vi "LCD Print.vi"(0 "Arduino Resource":T1, 5 "Data":string, 7 "Base (String)":T3(ring), 11 "error out":errorcluster) -> (4 "Arduino Resource":T1, 15 "error out":errorcluster)   [LabVIEW 2015, in "LabVIEW Interface for Arduino.lvlib"]
doc: "Prints data of the specified type to the LCD screen."
uses:
  <vilib>/LabVIEW Interface for Arduino/LabVIEW Interface for Arduino.lvlib
  <vilib>/LabVIEW Interface for Arduino/Type Defs/Arduino Resource.ctl
  <vilib>/LabVIEW Interface for Arduino/Type Defs/Board Type.ctl
  <vilib>/LabVIEW Interface for Arduino/Type Defs/Command.ctl
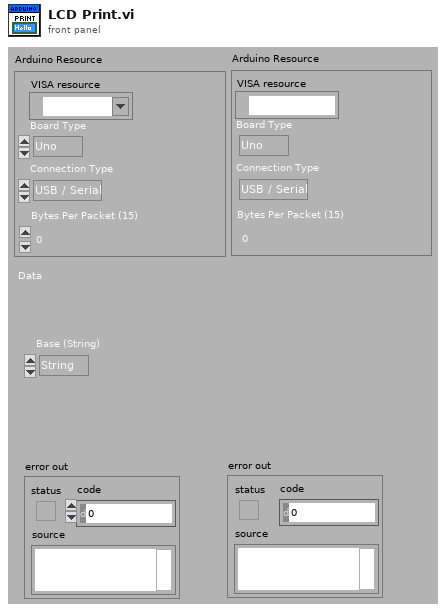
[diagram p1: front panel]
types:
  T1 = typedef "LabVIEW Interface for Arduino.lvlib/Arduino Resource.ctl" = cluster{"VISA resource":refnum<visa-resource-name>, "Board Type":T2, "Connection Type":enum8{"USB / Serial"}, "Bytes Per Packet (15)":u8}
  T2 = typedef "LabVIEW Interface for Arduino.lvlib/Board Type.ctl" = enum16{"Uno", "Dimuelanove w/Atmega 328", "Mega 2560"}
  T3 = enum8{"String", "Binary", "Decimal", "Octal", "Hexadecimal"}
  T4 = typedef "LabVIEW Interface for Arduino.lvlib/Command.ctl" = enum8{"setArduinoMode", "flushSerial", "setPinMode", "digitalWritePin", "digitalWritePort", "tone", "digitalReadPin", "digitalReadPort", "analogReadPin", "analogReadPort", "pwmWritePin", "pwmWritePort", "sevenSegment_Configure", "sevenSegment_Write", "I2C Init", "I2C Write", "I2C Read", "SPI Init", "SPI Set Bit Order", "SPI Set Clock Divider", "SPI Set Data Mode", "SPI Send / Receive", "SPI Close", "Servo Set Num Servos", "Servo Config Servo", "Servo Write Angle", "Servo Read Angle", "Servo Write Pulse Width", "Servo Read Pulse Width", "Servo Detach", "LCD Init", "LCD Set Size", "LCD Set Cursor Mode", "LCD Clear", "LCD Set Cursor Position", "LCD Print", "LCD Display Power", "LCD Scroll Display", "LCD Autoscroll", "LCD Print Direction", "LCD Create Custom Char", "LCD Print Custom Char", "contAcqOn", "contAcqOff", "getFirmwareVersion", "FiniteSampleStart"}
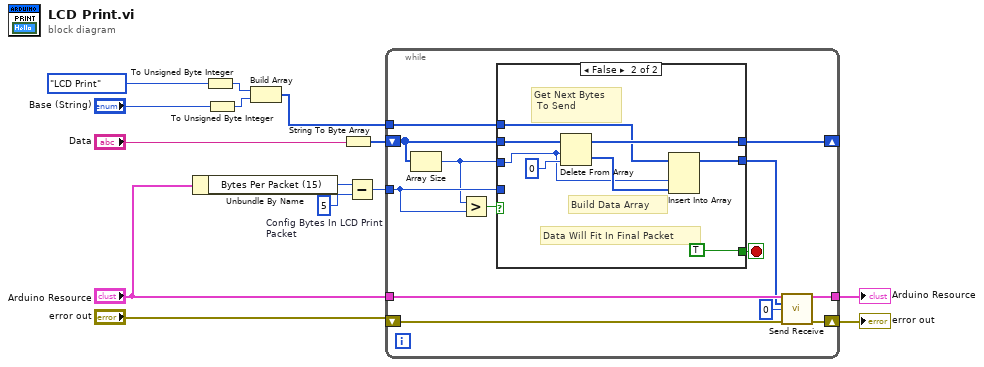
[diagram p0: block diagram]
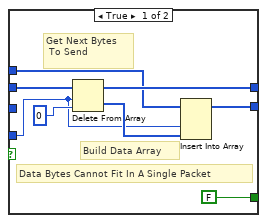
[diagram p2: hidden frame]
diagram:
  w6 = u8 5  # Config Bytes In LCD Print Packet
  n1 = Unbundle By Name("Arduino Resource") -> ("Bytes Per Packet (15)"=w2:u8)
  n2 = To Unsigned Byte Integer(number=Command."LCD Print" ("Command")) -> (unsigned 8bit integer=w10:u8)
  n3 = To Unsigned Byte Integer(number="Base (String)") -> (unsigned 8bit integer=w3:u8)
  n4 = Build Array(w10, w3) -> (w1:u8[])
  n5 = String To Byte Array(string="Data") -> (unsigned byte array=w5:u8[])
  n6 = Subtract(x=w2, y=w6) -> (x-y=w4:u8)
  n7 = while {
    tunnel: [w26] -> w13
    tunnel: "Arduino Resource" -> [w24]
    shift-right: [w27] -> w14
    shift-left: "error out" -> [w25]
    shift-right: [w22] -> _
    shift-left: w5 -> [w18]
    tunnel: w4 -> [w17]
    tunnel: w1 -> [w21]
    stop <- w15 stop-if-true
    n8 = Array Size(array=w18) -> (size(s)=w16:i32)
    n9 = Greater?(x=w16, y=w17) -> (0:w19:bool)
    n10 = case shown="False" w19 {
      tunnel: w18 -> [w35 w43]
      tunnel: w17 -> [w28 _]
      tunnel: [w33 w41] -> w22
      tunnel: w21 -> [w32 w40]
      tunnel: [w31 w39] -> w20
      tunnel: w16 -> [_ w36]
      tunnel: [FALSE TRUE] -> w15
      frame True {
        # "Data Bytes Cannot Fit In A Single Packet"
        # "Build Data Array"
        # "Get Next Bytes\n To Send"
        n11 = Delete From Array(array=w35, length=w28, index=0) -> (deleted portion=w29:u8[], array with subset deleted=w33:u8[])
        n12 = Insert Into Array(array=w32, new element #1=w28, new element #2=w29) -> (w31:u8[])  [unwired: 1 in]
      }
      frame False {
        # "Data Will Fit In Final Packet"
        # "Build Data Array"
        # "Get Next Bytes\n To Send"
        n13 = Delete From Array(array=w43, length=w36, index=0) -> (deleted portion=w37:u8[], array with subset deleted=w41:u8[])
        n14 = Insert Into Array(array=w40, new element #1=w36, new element #2=w37) -> (w39:u8[])  [unwired: 1 in]
      }
    }
    n15 = call <vilib>:"Send Receive.vi"("Arduino Resource"=w24, "Data"=w20, "Bytes To Read (0)"=u8 0, "error in"=w25) -> ("Arduino Resource"=w26:T1, "error out"=w27:errorcluster)  [unwired: 9 in, 1 out]
  }
  "error out" <- w14
  "Arduino Resource" <- w13
